vi "Config Load Sequence.vi"(8 "Sys Error In":errorcluster, 9 "Base Path":path=path "C:/Labview Code/System/Part Configuration", 10 "Station":string, 11 "Part Type":string) -> (0 "Sys Error Out":errorcluster, 1 "Sequence Name":string, 2 "Item Names":string[][](array[string]), 3 "Seqence Info":T1[](array[typedef]), 5 "Sequence Path":path)   [LabVIEW 2018]
uses:
  sequence/type defs/Sequence Info.ctl
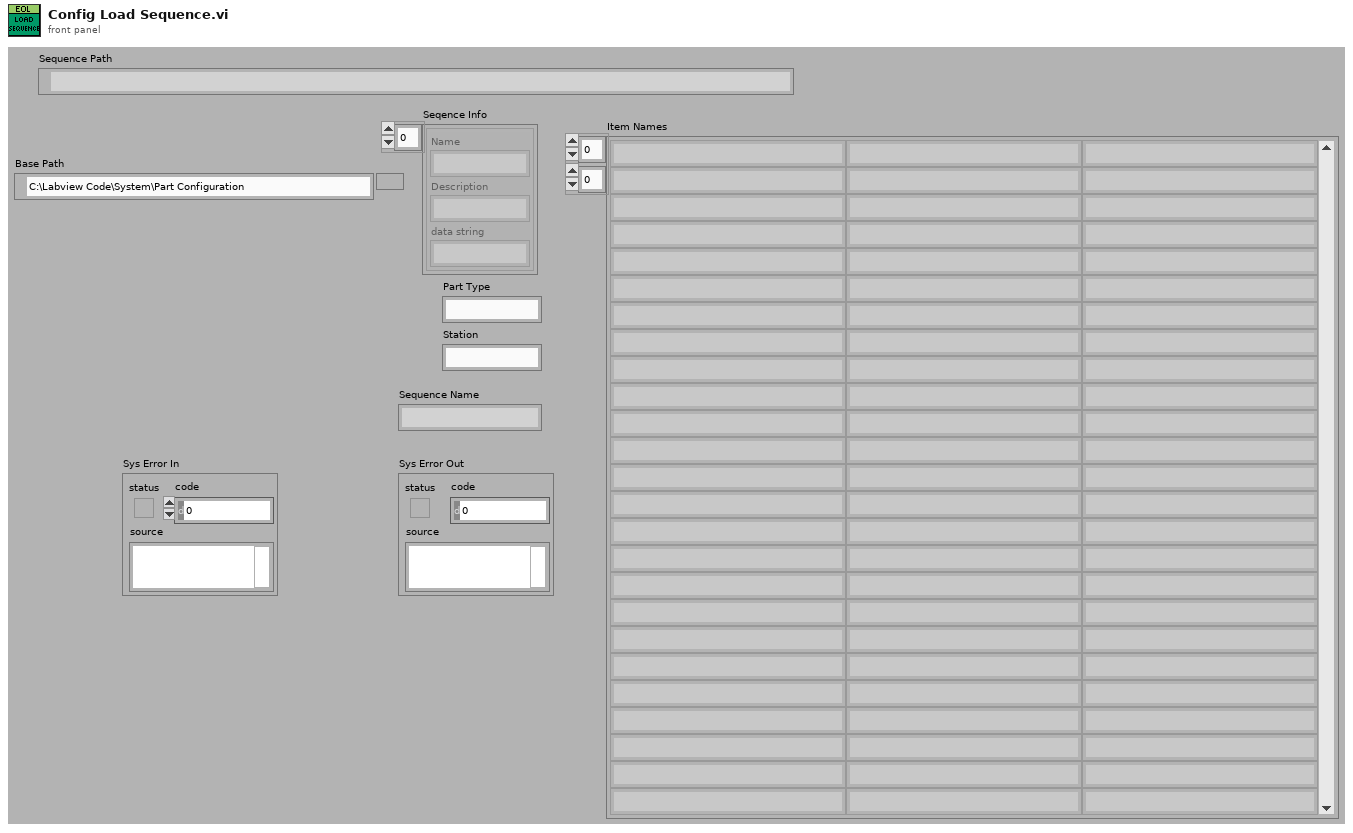
[diagram p1: front panel]
types:
  T1 = typedef "Sequence Info.ctl" = cluster{"Name":string, "Description":string, "data string":string}
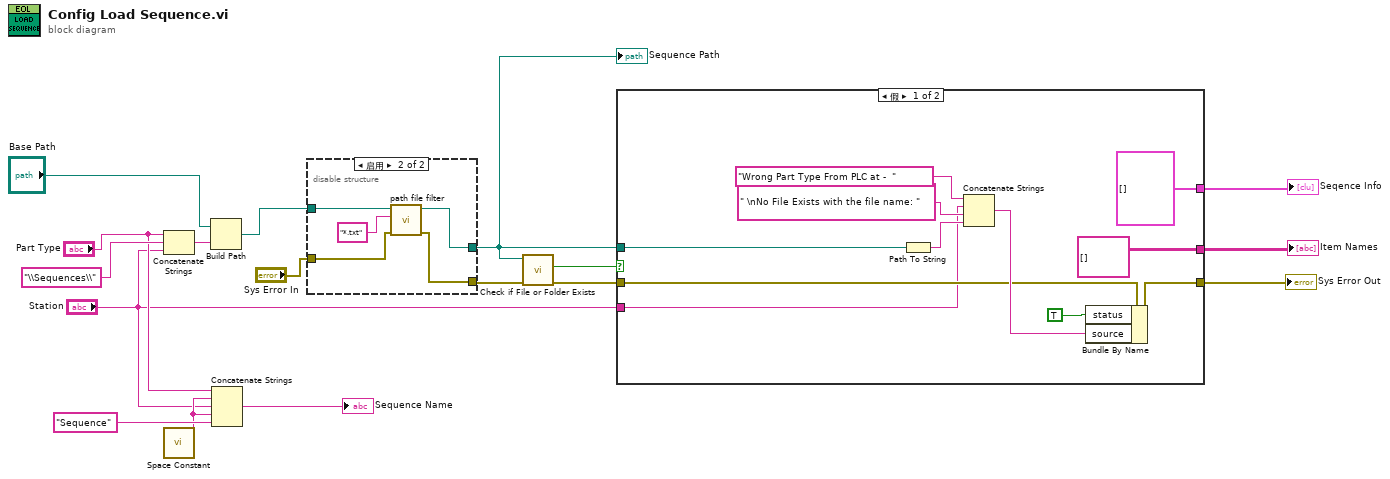
[diagram p0: block diagram]
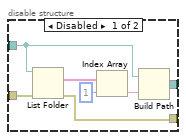
[diagram p2: hidden frame]
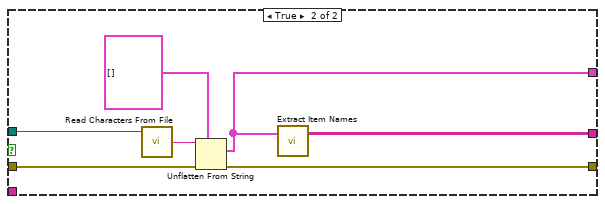
[diagram p3: hidden frame]
diagram:
  n1 = Concatenate Strings("Part Type", "\\Sequences\\" ("string"), "Station") -> (w17:string)
  n2 = call <vilib>:"Space Constant.vi"() -> ("String"=w7:string)
  n3 = Build Path(base path="Base Path", name or relative path=w17) -> (appended path=w5:path)
  n4 = Concatenate Strings("Part Type", w7, "Station", w7, "Sequence" ("string")) -> (→"Sequence Name":string)
  n5 = disable-structure shown="启用" {
    disable-tunnel: [w23 w25] -> w13
    disable-tunnel: w5 -> [w18 w28]
    disable-tunnel: "Sys Error In" -> [w22 w27]
    disable-tunnel: [w21 w26] -> w3
    frame Disabled {
      n6 = List Folder(path=w18, error in=w22) -> (filenames=w20:string[], error out=w21:errorcluster)  [unwired: 2 in, 2 out]
      n7 = Index Array(array=w20, index=1 ("索引")) -> (element=w24:string)
      n8 = Build Path(base path=w18, name or relative path=w24) -> (appended path=w23:path)
    }
    frame Enabled {
      n9 = call "path file filter.vi"("Sys Error In"=w27, "file type"="*.txt", "path"=w28) -> ("错误输出"=w26:errorcluster, "File path"=w25:path)  [unwired: 7 in]
    }
  }
  "Sequence Path" <- w13
  n10 = call <vilib>:"Check if File or Folder Exists.vi"("error in (no error)"=w3, "path"=w13) -> ("error out"=w2:errorcluster, "file or folder exists?"=w14:bool)  [unwired: 7 in, 1 out]
  n11 = case shown="假" w14 {
    tunnel: w13 -> [w36 w45]
    tunnel: [T1[] [] ("Seqence Info") w44] -> w12
    tunnel: [string[][] [] ("Item Names") w43] -> w11
    tunnel: w2 -> [w37 w42]
    tunnel: [w35 w41] -> w6
    tunnel: "Station" -> [w30 _]
    frame False {
      n12 = Path To String(path=w36) -> (string=w39:string)
      n13 = Concatenate Strings("Wrong Part Type From PLC at -  " ("string"), w30, " \nNo File Exists with the file name: " ("string"), w39) -> (w38:string)
      n14 = Bundle By Name(cluster=w37, "status"=TRUE, "source"=w38) -> (w35:errorcluster)
    }
    frame True {
      n15 = call <vilib>:"Read Characters From File.vi"("file path (dialog if empty)"=w45) -> ("character string"=w47:string)  [unwired: 5 in, 3 out]
      n16 = Unflatten From String(type=T1[] [] ("Seqence Info"), binary string=w47, error in (no error)=w42) -> (value=w44:T1[], error out=w41:errorcluster)  [unwired: 2 in, 1 out]
      n17 = call "Extract Item Names.vi"("Step Array"=w44) -> ("Item Names"=w43:string[][])  [unwired: 2 in]
    }
  }
  "Seqence Info" <- w12
  "Item Names" <- w11
  "Sys Error Out" <- w6
